vi "Test GUI.vi"() -> ()   [LabVIEW 2018]
doc: "Acoustic Test for EOL"
uses:
  Types/EnumType.ctl
  <vilib>/Utility/miscctls.llb/LVRowAndColumnTypeDef.ctl
  <vilib>/Utility/miscctls.llb/LVRowAndColumnUnsignedTypeDef.ctl
  <vilib>/Utility/error.llb/DialogType.ctl
  Supports/Global 1.vi
panel:
  out "1.6 part":bool
  out "1.7 part":bool
  out "ME79 MODEL":enum16{"E183362", "E180639", "E415025"}(ring)
  out "SN":u16
  in  "ZEBRA PRINT ME74":bool
  in  "Reset Conter 2":bool
  out "TARGET COUNTER":dbl
  in  "PLAN TARGET":dbl
  out "CounterFull 2":bool
  out "Buffer 2":u16
  out "Buffer":u16
  out "MIC 2":cluster{dbl[], dbl[]}[](graph)
  out "Test Data":string[][](table)
  out "MIC 1":cluster{dbl[], dbl[]}[](graph)
  in  "Change Model":bool
  in  "Alarm":u16
  out "Alarm Display":string
  out "MCError":bool
  out "Auto Running":bool
  out "CYCLE\nTIME":u16
  in  "Reset Conter":bool
  out "NG":dbl
  out "OK":dbl
  in  "BOX TARGET":dbl
  out "CounterFull":bool
  out "File Open Reference out":T1
  out "Test Error":bool
  out "Power OK":bool
  in  "Print":bool=TRUE
  out "LBL Data":T2
  in  "Cal Mic CH":bool
  out "AT Cond 2":bool
  out "AT Cond":bool
  in  "IAI Cal":bool
  in  "IAI Ret":bool
  in  "IAI Adv":bool
  out "Status":string
  in  "Calibrate":bool
  out "Connection":bool
  out "Stop":bool
  out "Start":bool
  out "Error":bool
  out "Fail":bool
  out "Pass":bool
  out "Done":bool
  out "Busy":bool
  out "Ready":bool
  in  "Channel":bool
  out "Model":bool
  in  "Start":bool
  in  "Mode":bool
  in  "Quit":bool
  out "Test Result":bool
  out "Test Running":bool
  # "MICROPHONE TEST EOL"
  # "TEST DATA"
  # "MANUAL CONTROL"
  # "BUFFER\nE180639"
  # "BUFFER\nE183362"
  # "Version 3.1 Build 20200630"
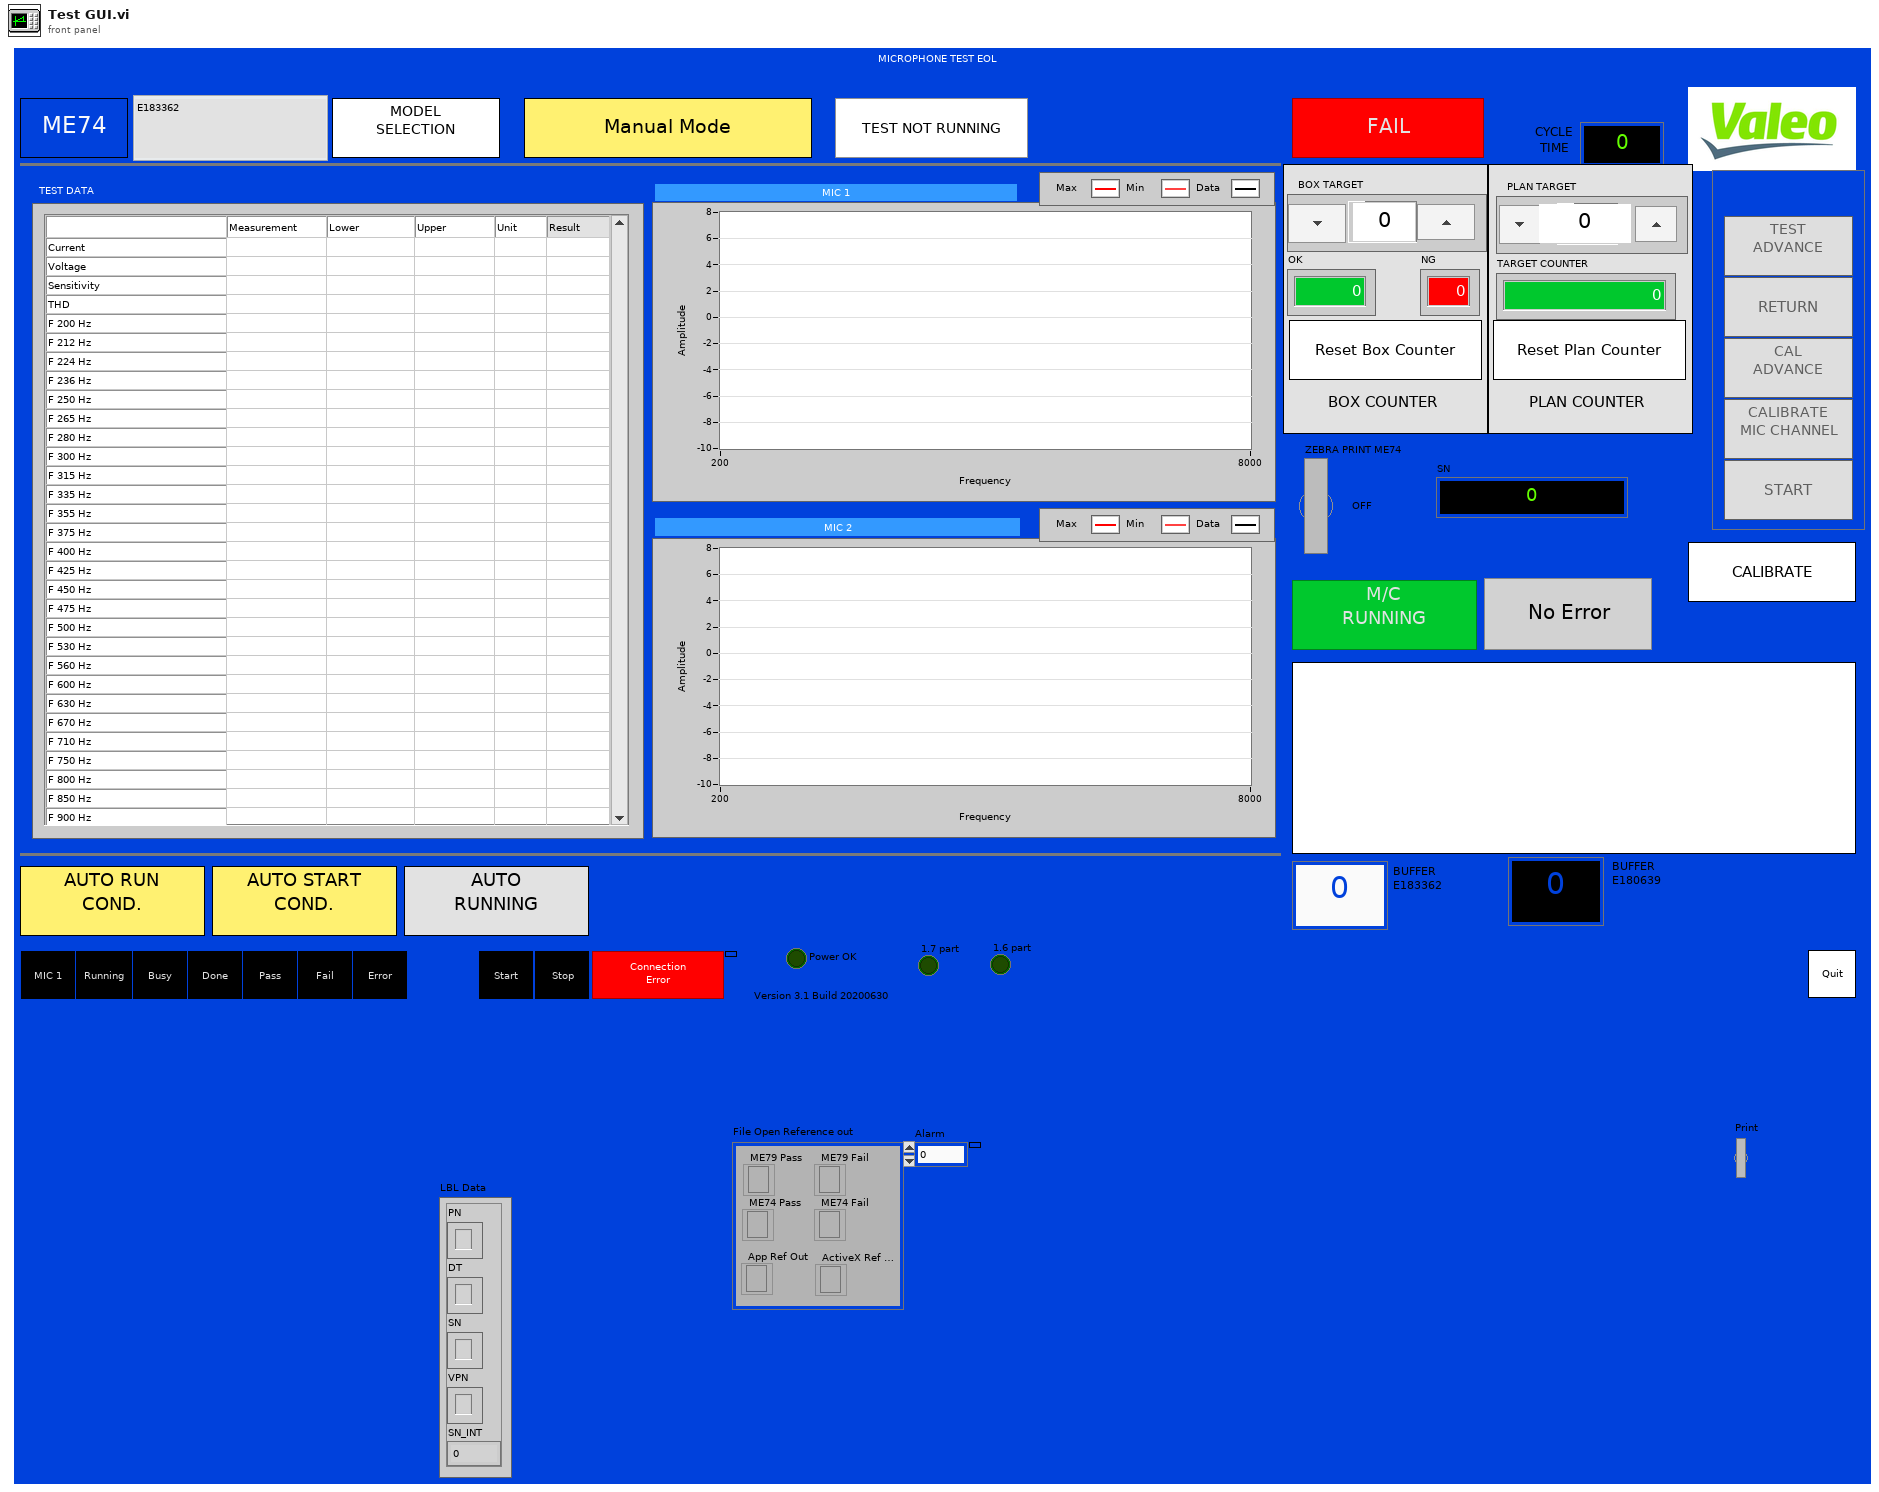
[diagram p1: front panel]
types:
  T1 = cluster{"ME79 Pass":refnum<k7>, "ME79 Fail":refnum<k7>, "ME74 Pass":refnum<k7>, "ME74 Fail":refnum<k7>, "App Ref Out":refnum<k7>, "ActiveX Ref Out":refnum<k7>}
  T2 = cluster{"PN":string, "DT":string, "SN":string, "VPN":string, "SN_INT":i32}
  T3 = typedef "EnumType.ctl" = enum16{"Initial", "Wait PLC Connect", "Ready", "Load and Init Config", "Power Supply On", "Freq Sweep 1", "Freq Sweep 2", "Power Supply Off", "Save Test Data", "Print Label", "Display Result", "Quit", "Calibration"}
  T4 = enum8{"Enabled", "Disabled", "Disabled and Grayed Out"}
  T5 = typedef "LVRowAndColumnTypeDef.ctl" = cluster{"Row":i32, "Column":i32}
  T6 = typedef "LVRowAndColumnUnsignedTypeDef.ctl" = cluster{"Row":u32, "Column":u32}
  T7 = typedef "LimitType.ctl" = cluster{"PSU":cluster{"Current Lower (mA)":dbl, "Current Upper (mA)":dbl, "Voltage Lower (V)":dbl, "Voltage Upper (V)":dbl}, "Mic":cluster{"Sensitivity (mV/Pa)":cluster{"Lower":dbl, "Upper":dbl}, "THD (%)":cluster{"Lower":dbl, "Upper":dbl}, "Freq Response":cluster{"Freq":dbl, "Upper":dbl, "Lower":dbl}[]}}
  T8 = typedef "ConfigurationType.ctl" = cluster{"PSU Setting":T9, "Sweep Settings":T10}
  T9 = typedef "SupplyConfig.ctl" = cluster{"Channel Name":string, "Source Delay (Sec)":dbl, "Measurement:Sense":i32, "voltage level":dbl, "voltage level range":dbl, "current limit":dbl, "current limit range":dbl, "resource name":refnum<k15>}
  T10 = typedef "Peiker_Stepped Sweep Settings.ctl" = cluster{"Input Settings":cluster{"IEPE min time to settle [s]":dbl, "Responce Channel Settings":cluster{"DSA response channel settings":T11, "response channel info":T12, "AI response settings":cluster{"response channel":tag, "max value [V]":dbl, "min value [V]":dbl, "terminal configuration":i32}}, "Stimulus Channel Settings":cluster{"AI stimulus settings":cluster{"stimulus channel":tag, "max value [V]":dbl, "min value [V]":dbl, "terminal configuration":i32}, "DSA stimulus channel settings":T11, "stimulus channel info":T12}}, "Output Settings":cluster{"AO source settings":cluster{"excitation channel":tag, "max value [V]":dbl, "min value [V]":dbl, "terminal configuration":i32}}}
  T11 = typedef "svc_DSA Channel Settings.ctl" = cluster{"coupling":i32, "enable IEPE excitation":bool, "IEPE current [mA]":dbl}
  T12 = typedef "svc_Channel Info.ctl" = cluster{"sensor sensitivity":dbl, "engineering units":T13, "dB reference":dbl, "custom label":string, "weighting filter":T14, "pregain":dbl}
  T13 = typedef "svc_Engineering Units Text Ring.ctl" = u16
  T14 = typedef "svc_Weighting Filter Text Ring.ctl" = u16
  T15 = cluster{"Label Data":string, "Label Data":string, "Label Data":string, "Label Data":string, "Cycle Time (ms)":i32}
  T16 = typedef "DialogType.ctl" = u16
  T17 = cluster{"frequency [Hz]":dbl[], "amplitude":dbl[]}
  T18 = cluster{string, "DT":string, "SN":string, "date/time string":string, "LINECODE":string, "NG CODE OUT":string}
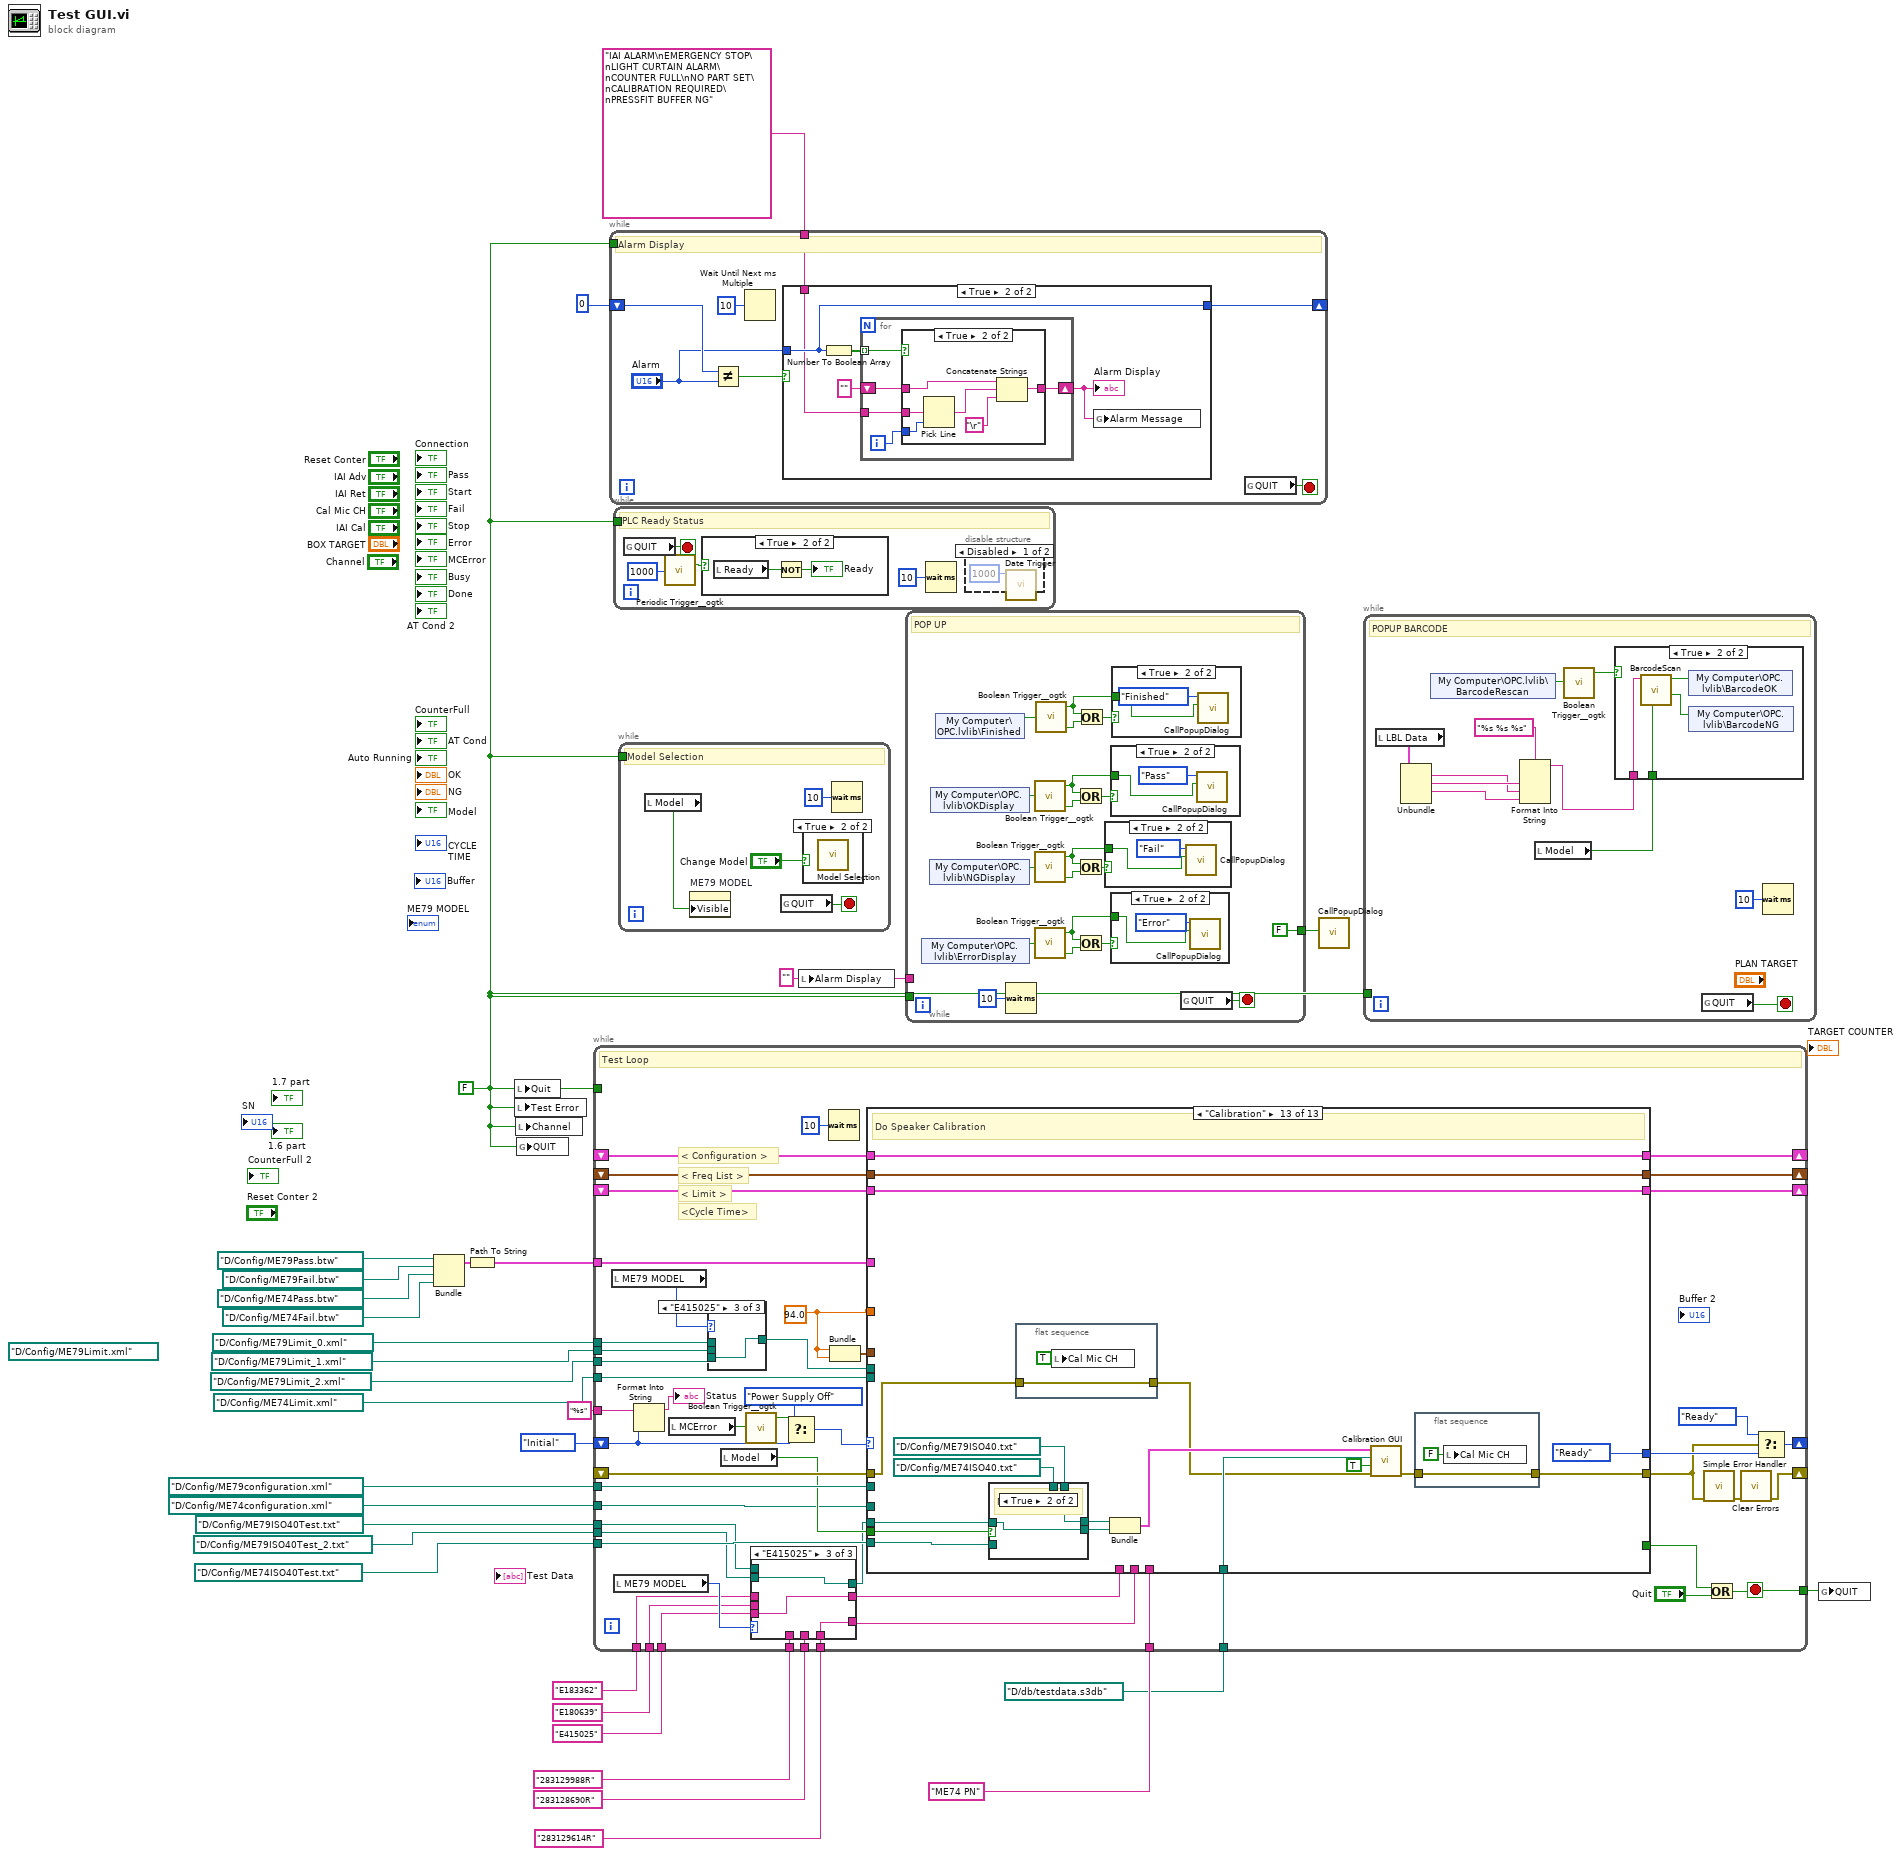
[diagram p0: block diagram]
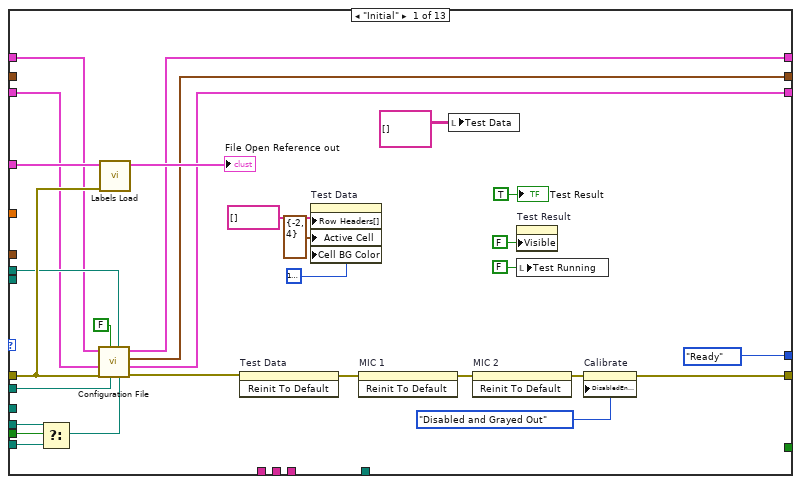
[diagram p16: hidden frame]
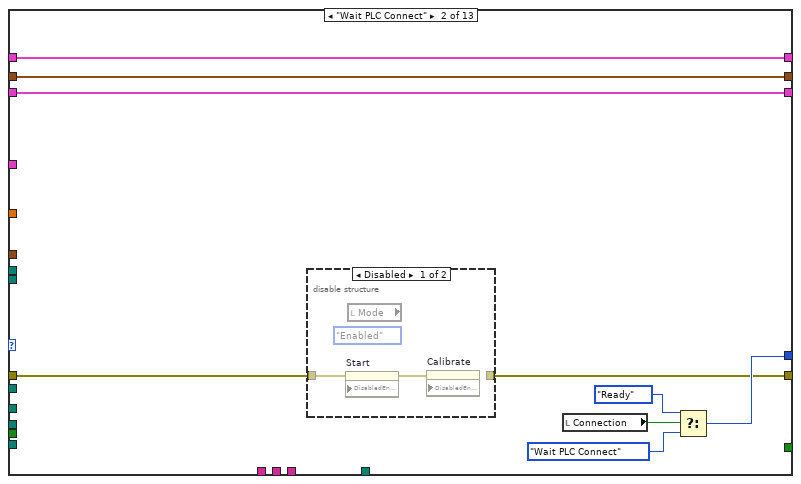
[diagram p17: hidden frame]
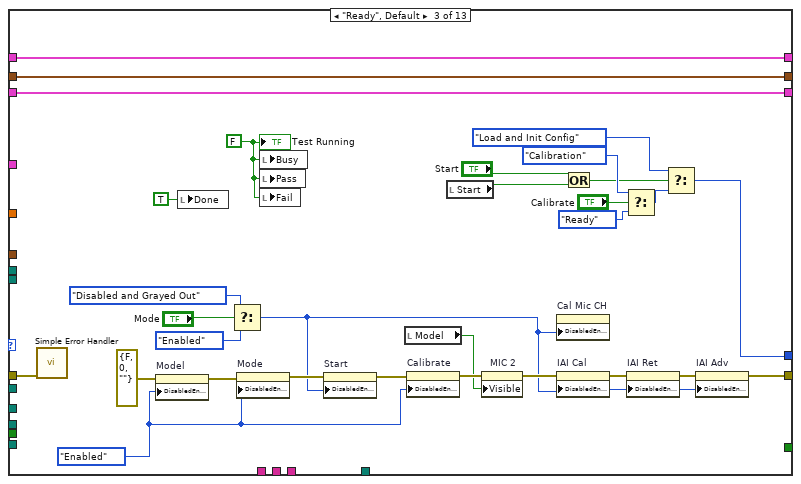
[diagram p19: hidden frame]
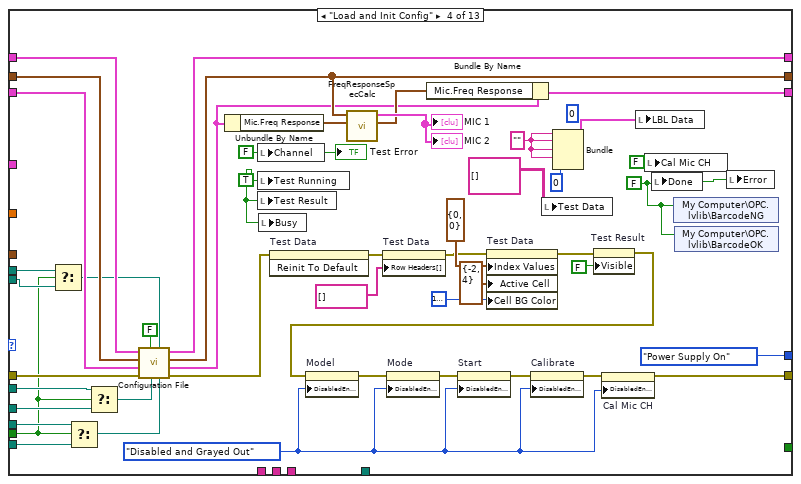
[diagram p20: hidden frame]
diagram:
  (unwired) path "D:/Config/ME79Limit.xml"
  w11 = ""
  w10 = FALSE ("Quit")
  n1 = Bundle(path "D:/Config/ME79Pass.btw", path "D:/Config/ME79Fail.btw", path "D:/Config/ME74Pass.btw", path "D:/Config/ME74Fail.btw") -> (w28:cluster{path, path, path, path})  [unwired: 1 in]
  n2 = Path To String(path=w28) -> (string=w29:cluster{string, string, string, string})
  n3 = local write "Quit"(w10) -> ()
  n4 = local write "Test Error"(w10) -> ()
  n5 = local write "Channel"(w10) -> ()
  n6 = global write "Global 1.vi" "QUIT"(w10) -> ()
  n7 = while {
    shift-right: [w71] -> _
    shift-left: EnumType."Initial" ("Enum") -> [w57]
    shift-right: [w69] -> _
    shift-left: _ -> [w81]
    tunnel: path "D:/Config/ME79configuration.xml" -> [w80]
    shift-right: [w79] -> _
    shift-left: _ -> [w78]
    shift-right: [w76] -> _
    shift-left: _ -> [w77]
    tunnel: path "D:/Config/ME79ISO40Test.txt" -> [w32]
    shift-right: [w74] -> _
    shift-left: _ -> [w75]
    tunnel: path "D:/Config/ME79Limit_0.xml" -> [w38]
    tunnel: path "D:/db/testdata.s3db" -> [w68]
    tunnel: path "D:/Config/ME74ISO40Test.txt" -> [w66]
    tunnel: w10 -> [_]
    tunnel: "ME74 PN" -> [w63]
    tunnel: w29 -> [w60]
    tunnel: "E183362" -> [w47]
    tunnel: "E180639" -> [w46]
    tunnel: "283129988R" -> [w42]
    tunnel: "283128690R" -> [w41]
    tunnel: path "D:/Config/ME74configuration.xml" -> [w53]
    tunnel: path "D:/Config/ME74Limit.xml" -> [w52]
    tunnel: "%s" ("format string") -> [w50]
    tunnel: [w49] -> w12
    tunnel: "E415025" -> [w45]
    tunnel: "283129614R" -> [w40]
    tunnel: path "D:/Config/ME79Limit_1.xml" -> [w37]
    tunnel: path "D:/Config/ME79Limit_2.xml" -> [w36]
    tunnel: path "D:/Config/ME79ISO40Test_2.txt" -> [w34]
    stop <- w49 stop-if-true
    w59 = 94.0 ("dB Reference")
    # "<Cycle Time>"
    # "< Limit >"
    # "< Freq List >"
    # "< Configuration >"
    # "Test Loop"
    n8 = local read "ME79 MODEL"() -> (w35:enum16{"E183362", "E180639", "E415025"})
    n9 = local read "ME79 MODEL"() -> (w48:enum16{"E183362", "E180639", "E415025"})
    n10 = Format Into String(format string=w50, w57) -> (resulting string=→"Status":string)  [unwired: 2 in, 1 out]
    n11 = local read "MCError"() -> (w55:bool)
    n12 = case shown="\"E415025\"" w35 {
      tunnel: [w83 w84 w85] -> w39
      tunnel: w38 -> [w83 _ _]
      tunnel: w37 -> [_ w84 _]
      tunnel: w36 -> [_ _ w85]
      frame "E183362", Default {
      }
      frame "E180639" {
      }
      frame "E415025" {
      }
    }
    n13 = local read "Model"() -> (w67:bool)
    n14 = call <userlib>:"Boolean Trigger__ogtk.vi"("Boolean Input"=w55) -> ("Rising Edge"=w54:bool)  [unwired: 1 in, 1 out]
    n15 = case shown="\"E415025\"" w48 {
      tunnel: w47 -> [w88 _ _]
      tunnel: w46 -> [_ w91 _]
      tunnel: w45 -> [_ _ w94]
      tunnel: [w88 w91 w94] -> w44
      tunnel: w42 -> [w87 _ _]
      tunnel: [w87 w90 w93] -> w43
      tunnel: w41 -> [_ w90 _]
      tunnel: w40 -> [_ _ w93]
      tunnel: w34 -> [_ _ w92]
      tunnel: [w86 w89 w92] -> w33
      tunnel: w32 -> [w86 w89 _]
      frame "E183362", Default {
      }
      frame "E180639" {
      }
      frame "E415025" {
      }
    }
    n16 = Select(t=EnumType."Power Supply Off" ("Enum"), s=w54, f=w57) -> (s? t:f=w56:T3)
    n17 = Wait (ms)(milliseconds to wait=u32 10) -> ()  [unwired: 1 out]
    n18 = Bundle("dB Reference"=w59, "dB Reference"=w59) -> (w62:cluster{"dB Reference":dbl, "dB Reference":dbl})  [unwired: 1 in]
    n19 = case shown="\"Calibration\"" w56 {
      tunnel: w81 -> [w108 w125 w162 w211 w238 w262 w294 w323 w354 w383 w417 w450 w457]
      tunnel: [w113 w124 w142 w179 w217 w242 w292 w325 w350 w397 w418 w450 w454] -> w61
      tunnel: [EnumType."Ready" ("Enum") w131 w157 EnumType."Power Supply On" ("Enum") w229 w245 EnumType."Power Supply Off" ("Enum") w315 EnumType."Print Label" ("Enum") EnumType."Display Result" ("Enum") EnumType."Ready" ("Enum") EnumType."Quit" ("Enum") EnumType."Ready" ("Enum")] -> w73
      tunnel: [_ _ _ _ _ _ _ _ _ _ _ TRUE _] -> w65
      tunnel: w80 -> [w106 _ _ w173 _ _ _ _ _ _ _ _ _]
      tunnel: [w99 w130 w165 w209 w222 w271 w303 w327 w357 w401 w422 w448 w465] -> w79
      tunnel: w78 -> [w98 w130 w165 w208 w222 w271 w303 w327 w357 w401 w422 w448 w465]
      tunnel: [w97 w129 w164 w186 w216 w248 w301 w329 w333 w400 w421 w447 w466] -> w76
      tunnel: w77 -> [_ w129 w164 w207 w216 w248 w301 w329 w333 w400 w421 w447 w466]
      tunnel: w33 -> [w104 _ _ w199 _ _ _ _ _ _ _ _ w462]
      tunnel: w75 -> [w95 w128 w163 w206 w215 w251 w282 w328 w356 w399 w420 w446 w467]
      tunnel: [w96 w128 w163 w202 w215 w251 w282 w328 w356 w399 w420 w446 w467] -> w74
      tunnel: w39 -> [w101 _ _ w171 _ _ _ _ _ _ _ _ _]
      tunnel: w68 -> [_ _ _ _ _ _ _ _ w353 _ _ _ w458]
      tunnel: w67 -> [w105 _ _ w169 _ w239 w275 _ w331 w375 _ _ w464]
      tunnel: w66 -> [w103 _ _ w198 _ _ _ _ _ _ _ _ w461]
      tunnel: w62 -> [_ _ _ _ _ w257 w288 _ _ _ _ _ _]
      tunnel: w59 -> [_ _ _ _ _ w256 w287 _ _ _ _ _ _]
      tunnel: w44 -> [_ _ _ _ _ _ _ _ w347 w377 _ _ _]
      tunnel: w63 -> [_ _ _ _ _ _ _ _ w346 _ _ _ _]
      tunnel: w60 -> [w110 _ _ _ _ _ _ _ _ _ _ _ _]
      tunnel: w43 -> [_ _ _ _ _ _ _ _ _ w378 _ _ _]
      tunnel: w53 -> [_ _ _ w174 _ _ _ _ _ _ _ _ _]
      tunnel: w52 -> [_ _ _ w170 _ _ _ _ _ _ _ _ _]
      frame "Initial" {
        n20 = Select(t=w104, s=w105, f=w103) -> (s? t:f=w102:path)
        n21 = call "Configuration File.vi"("Freq List File"=w102, "Limit File"=w101, "Configurtion File"=w106, "Mode (F-Read)"=FALSE, "Error In"=w108, "Limit"=w95, "Configuration"=w98) -> ("Error Out"=w107:errorcluster, "Limit Out"=w96:T7, "Freq List Out"=w97:cluster{"Freq":dbl, "Amp":dbl}[], "value"=w99:T8)  [unwired: 1 in]
        n22 = call "Labels Load.vi"("error in (no error)"=w108, "Labels"=w110) -> ("File Open Reference out"=→"File Open Reference out":T1)  [unwired: 8 in, 1 out]
        n23 = invoke on="Test Data" class="Tbl (strict)" method="Reinit To Default"(error in=w107) -> (error out=w121:errorcluster)  [unwired: 2 in, 2 out]
        n24 = property on="Test Data" class="Tbl (strict)"("Row Headers[]"=string[] [], "Active Cell"=T5 {"Row"=-2, "Column"=4} ("Active Cell:Active Cell"), "Cell BG Color"=u32 16777225) -> ()  [unwired: 2 in, 2 out]
        n25 = invoke on="MIC 1" class="XYGraph (strict)" method="Reinit To Default"(error in=w121) -> (error out=w120:errorcluster)  [unwired: 2 in, 2 out]
        n26 = local write "Test Data"(string[][] []) -> ()
        n27 = invoke on="MIC 2" class="XYGraph (strict)" method="Reinit To Default"(error in=w120) -> (error out=w114:errorcluster)  [unwired: 2 in, 2 out]
        n28 = property on="Test Result" class="Bool (strict)"("Visible"=FALSE) -> ()  [unwired: 2 in, 2 out]
        n29 = local write "Test Running"(FALSE ("Test Running")) -> ()
        n30 = property on="Calibrate" class="Bool"(error in=w114, "DisabledEnum"=T4."Disabled and Grayed Out" ("Disabled")) -> (error out=w113:errorcluster)  [unwired: 1 in, 1 out]
        "Test Result" <- TRUE ("Test Pass")
      }
      frame "Wait PLC Connect" {
        n31 = disable-structure shown="Disabled" {
          disable-tunnel: w125 -> [w134 w135]
          disable-tunnel: [_ w135] -> w124
          frame Disabled {
            (unwired) T4."Enabled" ("Disabled")
            n32 = property on="Start" class="Bool (strict)" props=["DisabledEnum"](error in=w134) -> (error out=w133:errorcluster)  [unwired: 2 in, 1 out]
            n33 = local read "Mode"() -> ()  [unwired: 1 out]
            n34 = property on="Calibrate" class="Bool" props=["DisabledEnum"](error in=w133) -> ()  [unwired: 2 in, 2 out]
          }
          frame Enabled {
          }
        }
        n35 = local read "Connection"() -> (w132:bool)
        n36 = Select(t=EnumType."Ready" ("Enum"), s=w132, f=EnumType."Wait PLC Connect" ("Enum")) -> (s? t:f=w131:T3)
      }
      frame "Ready", Default {
        w147 = T4."Enabled" ("Disabled")
        w139 = FALSE ("Test Running")
        n37 = call <vilib>:"Simple Error Handler.vi"("error in (no error)"=w162) -> ()  [unwired: 4 in, 5 out]
        n38 = property on="Model" class="Bool (strict)"(error in=errorcluster {"status"=FALSE, "code"=0, "source"=""} ("Error Out"), "DisabledEnum"=w147) -> (error out=w151:errorcluster)  [unwired: 1 in, 1 out]
        n39 = local write "Done"(TRUE ("Done")) -> ()
        n40 = Select(t=T4."Disabled and Grayed Out" ("Disabled"), s="Mode", f=T4."Enabled" ("Disabled")) -> (s? t:f=w138:T4)
        n41 = property on="Mode" class="Bool (strict)"(error in=w151, "DisabledEnum"=w147) -> (error out=w150:errorcluster)  [unwired: 1 in, 1 out]
        n42 = local write "Busy"(w139) -> ()
        n43 = local write "Pass"(w139) -> ()
        n44 = local write "Fail"(w139) -> ()
        n45 = property on="Start" class="Bool (strict)"(error in=w150, "DisabledEnum"=w138) -> (error out=w148:errorcluster)  [unwired: 1 in, 1 out]
        n46 = local read "Model"() -> (w136:bool)
        n47 = property on="Calibrate" class="Bool"(error in=w148, "DisabledEnum"=w147) -> (error out=w146:errorcluster)  [unwired: 1 in, 1 out]
        n48 = local read "Start"() -> (w137:bool)
        n49 = property on="MIC 2" class="XYGraph (strict)"(error in=w146, "Visible"=w136) -> (error out=w143:errorcluster)  [unwired: 1 in, 1 out]
        n50 = property on="Cal Mic CH" class="Bool (strict)"("DisabledEnum"=w138) -> ()  [unwired: 2 in, 2 out]
        n51 = property on="IAI Cal" class="Bool (strict)"(error in=w143, "DisabledEnum"=w138) -> (error out=w145:errorcluster)  [unwired: 1 in, 1 out]
        n52 = Or(x="Start", y=w137) -> (x .or. y?=w153:bool)
        n53 = Select(t=EnumType."Calibration" ("Enum"), s="Calibrate", f=EnumType."Ready" ("Enum")) -> (s? t:f=w158:T3)
        n54 = property on="IAI Ret" class="Bool (strict)"(error in=w145, "DisabledEnum"=w138) -> (error out=w144:errorcluster)  [unwired: 1 in, 1 out]
        n55 = Select(t=EnumType."Load and Init Config" ("Enum"), s=w153, f=w158) -> (s? t:f=w157:T3)
        n56 = property on="IAI Adv" class="Bool (strict)"(error in=w144, "DisabledEnum"=w138) -> (error out=w142:errorcluster)  [unwired: 1 in, 1 out]
        "Test Running" <- w139
      }
      frame "Load and Init Config" {
        w175 = "" ("Label Data")
        w167 = FALSE ("Done")
        (unwired) 0 ("Cycle Time (ms)")
        w176 = FALSE ("Channel")
        w182 = TRUE ("Test Running")
        w178 = T4."Disabled and Grayed Out" ("Disabled")
        n57 = Select(t=w171, s=w169, f=w170) -> (s? t:f=w168:path)
        n58 = Select(t=w199, s=w169, f=w198) -> (s? t:f=w197:path)
        n59 = Select(t=w173, s=w169, f=w174) -> (s? t:f=w172:path)
        n60 = call "Configuration File.vi"("Freq List File"=w197, "Limit File"=w168, "Configurtion File"=w172, "Mode (F-Read)"=FALSE, "Error In"=w211, "Limit"=w206, "Freq List In"=w207, "Configuration"=w208) -> ("Error Out"=w194:errorcluster, "Limit Out"=w185:T7, "Freq List Out"=w186:cluster{"Freq":dbl, "Amp":dbl}[], "value"=w209:T8)
        n61 = Unbundle By Name(w185) -> ("Mic.Freq Response"=w205:cluster{"Freq":dbl, "Upper":dbl, "Lower":dbl}[])
        n62 = local write "Channel"(w176) -> ()
        n63 = local write "Test Running"(w182) -> ()
        n64 = local write "Test Result"(w182) -> ()
        n65 = local write "Busy"(w182) -> ()
        n66 = invoke on="Test Data" class="Tbl (strict)" method="Reinit To Default"(error in=w194) -> (error out=w200:errorcluster)  [unwired: 2 in, 2 out]
        n67 = call "FreqResponseSpecCalc.vi"("Freq Response Spec In"=w205, "Freq List In"=w186) -> ("All Freq Spec Out"=w203:cluster{"Freq":dbl, "Upper":dbl, "Lower":dbl}[], "XY Graph"=→"MIC 1" →"MIC 2":cluster{dbl[], dbl[]}[])  [unwired: 8 in]
        n68 = property on="Test Data" class="Tbl (strict)"(error in=w200, "Row Headers[]"=string[] [] ("Row Header Strings[]")) -> (error out=w195:errorcluster)  [unwired: 1 in, 1 out]
        n69 = Bundle By Name(cluster=w185, "Mic.Freq Response"=w203) -> (w202:T7)
        n70 = property on="Test Data" class="Tbl (strict)"(error in=w195, "Index Values"=T6 {"Row"=0, "Column"=0}, "Active Cell"=T5 {"Row"=-2, "Column"=4} ("Active Cell:Active Cell"), "Cell BG Color"=u32 16777225) -> (error out=w184:errorcluster)  [unwired: 1 in, 1 out]
        n71 = local write "Test Data"(string[][] []) -> ()
        n72 = Bundle("Label Data"=w175, "Label Data"=w175, "Label Data"=w175, "Label Data"=w175, "Cycle Time (ms)"=0) -> (w177:T15)  [unwired: 1 in]
        n73 = property on="Test Result" class="Bool (strict)"(error in=w184, "Visible"=FALSE) -> (error out=w183:errorcluster)  [unwired: 1 in, 1 out]
        n74 = property on="Model" class="Bool (strict)"(error in=w183, "DisabledEnum"=w178) -> (error out=w192:errorcluster)  [unwired: 1 in, 1 out]
        n75 = property on="Mode" class="Bool (strict)"(error in=w192, "DisabledEnum"=w178) -> (error out=w191:errorcluster)  [unwired: 1 in, 1 out]
        n76 = property on="Start" class="Bool (strict)"(error in=w191, "DisabledEnum"=w178) -> (error out=w188:errorcluster)  [unwired: 1 in, 1 out]
        n77 = property on="Calibrate" class="Bool"(error in=w188, "DisabledEnum"=w178) -> (error out=w180:errorcluster)  [unwired: 1 in, 1 out]
        n78 = property on="Cal Mic CH" class="Bool (strict)"(error in=w180, "DisabledEnum"=w178) -> (error out=w179:errorcluster)  [unwired: 1 in, 1 out]
        n79 = local write "LBL Data"(w177) -> ()
        n80 = local write "Cal Mic CH"(FALSE ("IAI Cal 2")) -> ()
        n81 = local write "Done"(w167) -> ()
        n82 = shared-variable "My Computer\\OPC.lvlib\\BarcodeNG"(w167) -> ()  [unwired: 1 in, 1 out]
        n83 = shared-variable "My Computer\\OPC.lvlib\\BarcodeOK"(w167) -> ()  [unwired: 1 in, 1 out]
        n84 = local write "Error"(w167) -> ()
        "Test Error" <- w176
      }
      frame "Power Supply On" {
        n85 = Unbundle By Name(w222) -> ("PSU Setting"=w221:T9)
        n86 = Unbundle By Name(w215) -> ("PSU.Current Upper (mA)"=w237:dbl, "PSU.Current Lower (mA)"=w236:dbl, "PSU.Voltage Upper (V)"=w235:dbl, "PSU.Voltage Lower (V)"=w234:dbl)
        n87 = call "PSU ON.vi"("Error In"=w238, "PSU Setting"=w221) -> ("Error Out"=w228:errorcluster, "Current Result (mA)"=w227:dbl, "Volt Result"=w226:dbl)  [unwired: 6 in, 1 out]
        n88 = local read "Test Result"() -> (w224:bool)
        n89 = control-ref of="Test Data"() -> (w219:refnum<vi>)
        n90 = Build Array(w227, w226) -> (w225:dbl[])
        n91 = In Range and Coerce(upper limit=w237, x=w227, lower limit=w236) -> (In Range?=w233:bool)  [unwired: 1 out]
        n92 = In Range and Coerce(upper limit=w235, x=w226, lower limit=w234) -> (In Range?=w232:bool)  [unwired: 1 out]
        n93 = call "Update Test Data Table.vi"("Enum"=enum16{"PSU", "Mic"}."PSU", "Prev Result in"=w224, "Error In"=w228, "Test Data In"=w225, "Limit In"=w215, "Test Data ref in"=w219) -> ("Error Out"=w220:errorcluster, "Latest Result Out"=w214:bool)  [unwired: 4 in]
        n94 = And(x=w233, y=w232) -> (x .and. y?=w213:bool)
        "Power OK" <- w213
        n95 = local write "Test Result"(w214) -> ()
        n96 = call "Table Result Color.vi"("Error In"=w220, "Result Column"=4, "Table Ref"=w219) -> ("Error Out"=w217:errorcluster)  [unwired: 8 in]
        n97 = Select(t=EnumType."Freq Sweep 1" ("Enum"), s=w213, f=EnumType."Power Supply Off" ("Enum")) -> (s? t:f=w229:T3)
      }
      frame "Freq Sweep 1" {
        w240 = T16 0 items=["no dialog", "OK message", "continue or stop message", "OK message + warnings", "continue/stop + warnings"] ("type of dialog (OK msg:1)")
        n98 = stacked-sequence {
          tunnel: w262 -> [_ w274]
          tunnel: [_ w273] -> w261
          frame #0 {
            n99 = local write "Channel"(FALSE) -> ()
          }
          frame #1 {
            n100 = call "Time Delay2"("error in (no error)"=w274) -> ("error out"=w273:errorcluster)  [unwired: 10 in]
          }
        }
        n101 = Unbundle By Name(w251) -> ("Mic.Freq Response"=w250:cluster{"Freq":dbl, "Upper":dbl, "Lower":dbl}[])
        n102 = Unbundle By Name(w271) -> ("Sweep Settings"=w270:T10)
        n103 = local read "Test Result"() -> (w265:bool)
        n104 = local read "MIC 1"() -> (w254:cluster{dbl[], dbl[]}[])
        n105 = call "Single Mic Test.vi"("Peiker_Stepped Sweep Settings"=w270, "Freq Response Limit"=w250, "frequency list Input"=w248, "Error In"=w261, "Test Level"=w257, "Model (T-79)"=w239, "dB Reference"=w256, "String"="SW1.txt") -> ("Processed Freq Response"=w253:T17, "Test Result Out"=w266:dbl[], "Error Out"=w264:errorcluster)  [unwired: 4 in, 1 out]
        n106 = Insert Into Array(array=w254, new element=w253) -> (w252:cluster{dbl[], dbl[]}[])  [unwired: 1 in]
        n107 = control-ref of="Test Data"() -> (w259:refnum<vi>)
        n108 = call "Update Test Data Table.vi"("Enum"=enum16{"PSU", "Mic"}."Mic", "Prev Result in"=w265, "Error In"=w264, "Test Data In"=w266, "Limit In"=w251, "Test Data ref in"=w259) -> ("Error Out"=w260:errorcluster, "Latest Result Out"=w249:bool)  [unwired: 4 in]
        n109 = local write "MIC 1"(w252) -> ()
        n110 = call "Table Result Color.vi"("Error In"=w260, "Result Column"=4, "Table Ref"=w259) -> ("Error Out"=w244:errorcluster)  [unwired: 8 in]
        n111 = local write "Test Result"(w249) -> ()
        n112 = call <vilib>:"Simple Error Handler.vi"("type of dialog (OK msg:1)"=w240, "error in (no error)"=w244) -> ("error?"=w241:bool, "error out"=w243:errorcluster)  [unwired: 3 in, 3 out]
        n113 = local read "Model"() -> (w269:bool)
        n114 = local write "Test Error"(w241) -> ()
        n115 = call <userlib>:"Clear All Errors__ogtk.vi"("Error In"=w243) -> ("Error Out"=w242:errorcluster)  [unwired: 3 in]
        n116 = Select(t=EnumType."Freq Sweep 2" ("Enum"), s=w269, f=EnumType."Power Supply Off" ("Enum")) -> (s? t:f=w246:T3)
        n117 = local write "Error"(w241) -> ()
        n118 = Select(t=EnumType."Power Supply Off" ("Enum"), s=w244, f=w246) -> (s? t:f=w245:T3)
      }
      frame "Freq Sweep 2" {
        w276 = T16 0 items=["no dialog", "OK message", "continue or stop message", "OK message + warnings", "continue/stop + warnings"] ("type of dialog (OK msg:1)")
        n119 = stacked-sequence {
          tunnel: w294 -> [_ w310]
          tunnel: [_ w309] -> w293
          frame #0 {
            n120 = local write "Channel"(TRUE) -> ()
          }
          frame #1 {
            n121 = call "Time Delay"("error in (no error)"=w310) -> ("error out"=w309:errorcluster)  [unwired: 10 in]
          }
        }
        n122 = Unbundle By Name(w303) -> ("Sweep Settings"=w302:T10)
        n123 = Unbundle By Name(w282) -> ("Mic.Freq Response"=w281:cluster{"Freq":dbl, "Upper":dbl, "Lower":dbl}[])
        n124 = local read "Test Result"() -> (w296:bool)
        n125 = local read "MIC 2"() -> (w285:cluster{dbl[], dbl[]}[])
        n126 = call "Single Mic Test.vi"("Peiker_Stepped Sweep Settings"=w302, "Freq Response Limit"=w281, "frequency list Input"=w301, "Error In"=w293, "Test Level"=w288, "Model (T-79)"=w275, "dB Reference"=w287, "String"="SW2.txt") -> ("Processed Freq Response"=w284:T17, "Test Result Out"=w297:dbl[], "Error Out"=w298:errorcluster)  [unwired: 4 in, 1 out]
        n127 = control-ref of="Test Data"() -> (w291:refnum<vi>)
        n128 = Insert Into Array(array=w285, new element=w284) -> (w283:cluster{dbl[], dbl[]}[])  [unwired: 1 in]
        n129 = call "Update Test Data Table.vi"("Enum"=enum16{"PSU", "Mic"}."Mic", "Prev Result in"=w296, "Error In"=w298, "Test Data In"=w297, "Limit In"=w282, "Test Data ref in"=w291) -> ("Error Out"=w289:errorcluster, "Latest Result Out"=w295:bool)  [unwired: 4 in]
        n130 = local write "MIC 2"(w283) -> ()
        n131 = call "Table Result Color.vi"("Error In"=w289, "Result Column"=4, "Table Ref"=w291) -> ("Error Out"=w280:errorcluster)  [unwired: 8 in]
        n132 = local write "Test Result"(w295) -> ()
        n133 = call <vilib>:"Simple Error Handler.vi"("type of dialog (OK msg:1)"=w276, "error in (no error)"=w280) -> ("error?"=w277:bool, "error out"=w279:errorcluster)  [unwired: 3 in, 3 out]
        n134 = call <userlib>:"Clear All Errors__ogtk.vi"("Error In"=w279) -> ("Error Out"=w278:errorcluster)  [unwired: 3 in]
        n135 = local write "Test Error"(w277) -> ()
        n136 = stacked-sequence {
          tunnel: w278 -> [_ w307]
          tunnel: [_ w306] -> w292
          frame #0 {
            n137 = local write "Channel"(FALSE) -> ()
          }
          frame #1 {
            n138 = call "Time Delay3"("error in (no error)"=w307, "Delay Time (s)"=0.2) -> ("error out"=w306:errorcluster)  [unwired: 9 in]
          }
        }
        n139 = local write "Error"(w277) -> ()
      }
      frame "Power Supply Off" {
        n140 = Unbundle By Name(w327) -> ("PSU Setting.resource name"=w311:refnum<k15>)
        n141 = property on="Test Result" class="Bool (strict)"(error in=w323, "Visible"=TRUE) -> (error out=w322:errorcluster)  [unwired: 1 in, 1 out]
        n142 = control-ref of="Test Data"() -> (w319:refnum<vi>)
        n143 = call "Reset_Power_Supply.vi"("error in (no error)"=errorcluster {"status"=FALSE, "code"=0, "source"=""}, "resource name"=w311) -> ("error out"=w321:errorcluster)  [unwired: 9 in]
        n144 = call "Table Result Color.vi"("Error In"=w321, "Result Column"=4, "Table Ref"=w319) -> ("Error Out"=w320:errorcluster)  [unwired: 8 in]
        n145 = Merge Errors(w322, w320) -> (w325:errorcluster)
        n146 = local read "MCError"() -> (w314:bool)
        n147 = local read "Test Error"() -> (w313:bool)
        n148 = Or(x=w314, y=w313) -> (x .or. y?=w312:bool)
        n149 = Select(t=EnumType."Display Result" ("Enum"), s=w312, f=EnumType."Save Test Data" ("Enum")) -> (s? t:f=w315:T3)
      }
      frame "Save Test Data" {
        (unwired) string[] [] ("f")
        n150 = local read "Test Data"() -> (w343:string[][])
        n151 = for {
          tunnel: w333 -> [_] mode=indexing
          tunnel: ["0"] -> w330 mode=indexing
        }
        n152 = Index Array(array=w343, index (col)=0 ("disabled index (col)")) -> (element=w339:string[])  [unwired: 1 in]
        n153 = local read "Model"() -> (w348:bool)
        n154 = Index Array(array=w339) -> (element #1=w342:string, element #2=w341:string)  [unwired: 2 in]
        n155 = case shown="True" w331 {
          tunnel: "0" -> [w363 w368]
          tunnel: w342 -> [w362 w367]
          tunnel: w341 -> [w361 w366]
          tunnel: [w360 w365] -> w338
          tunnel: w330 -> [w359 w364]
          tunnel: w330 -> [w358 _]
          frame True {
            n156 = Build Array (concatenate)(w362, w361, w363, w363, w359, w363, w363, w358) -> (w360:string[])
          }
          frame False {
            n157 = Build Array (concatenate)(w367, w366, w368, w368, w364) -> (w365:string[])
          }
        }
        n158 = local read "Power OK"() -> (w340:bool)
        n159 = Select(t=w339, s=w340, f=w338) -> (s? t:f=w332:string[])
        n160 = local read "Test Result"() -> (w336:bool)
        n161 = Select(t=w347, s=w348, f=w346) -> (s? t:f=w345:string)
        n162 = call "Data Logger.vi"("PN In"=w345, "Test Result?"=w336, "Error In"=w354, "DB File"=w353, "Model (F-ME74)"=w348, "Test Data In"=w332) -> ("Error Out"=w351:errorcluster, "LBL Data"=w335:T2)  [unwired: 3 in, 1 out]
        "LBL Data" <- w335
        n163 = Not(x=w336) -> (.not. x?=w337:bool)
        n164 = local write "Pass"(w336) -> ()
        n165 = Unbundle By Name(w335) -> ("SN_INT"=w334:i32)
        n166 = local write "Fail"(w337) -> ()
        n167 = control-ref of="Test Data"() -> (w349:refnum<vi>)
        n168 = local write "SN"(w334) -> ()
        n169 = call "Log File.vi"("Error In"=w351, "Model (F-ME74)"=w348, "Test Data table"=w349) -> ("Error Out"=w350:errorcluster)  [unwired: 8 in]
      }
      frame "Print Label" {
        n170 = local read "Test Data"() -> (w381:string[][])
        n171 = local read "LBL Data"() -> (w379:T2)
        n172 = Get Date/Time In Seconds() -> (seconds since 1Jan1904=w393:timestamp)
        n173 = Format Date/Time String(time format string (%c)="%H%M", seconds (now)=w393) -> (date/time string=w391:string)  [unwired: 1 in]
        n174 = call "NGCode.vi"("error in (no error)"=w383, "Test Data"=w381) -> ("error out"=w382:errorcluster, "NG CODE OUT"=w380:string)  [unwired: 8 in]
        n175 = Unbundle(w379) -> ("DT"=w396:string, "SN"=w395:string)  [unwired: 3 out]
        n176 = local read "File Open Reference out"() -> (w394:T1)
        n177 = local read "Test Result"() -> (w386:bool)
        n178 = Bundle(w377, "DT"=w396, "SN"=w395, "date/time string"=w391, "LINECODE"="1", "NG CODE OUT"=w380) -> (w389:T18)  [unwired: 1 in]
        n179 = Bundle By Name(cluster=w379, "PN"=w378, "VPN"=w377) -> (w388:T2)
        n180 = Select(t=TRUE, s=w375, f="ZEBRA PRINT ME74") -> (s? t:f=w370:bool)
        n181 = And(x="Print", y=w370) -> (x .and. y?=w371:bool)
        n182 = case shown="True" w371 {
          tunnel: w382 -> [w404 w413]
          tunnel: [w404 w412] -> w397
          tunnel: w394 -> [_ w411]
          tunnel: w389 -> [_ w410]
          tunnel: w388 -> [_ w409]
          tunnel: w386 -> [_ w408]
          tunnel: w375 -> [_ w407]
          tunnel: [FALSE FALSE] -> w385
          tunnel: [TRUE TRUE] -> w384
          frame False {
          }
          frame True {
            n183 = call "Label PrintOut.vi"("Model (F-ME74)"=w407, "Label Print Pass/Fail (F-Fail)"=w408, "error in (no error)"=w413, "Fail Data"=w410, "Pass Data"=w409, "Labels Reference In"=w411) -> ("error out"=w412:errorcluster)  [unwired: 5 in]
          }
        }
        n184 = Bundle By Name(cluster=w379, "PN"=w378, "VPN"=w377) -> (w376:T2)
        n185 = local write "LBL Data"(w376) -> ()
        n186 = local write "Done"(w384) -> ()
        n187 = local write "Busy"(w385) -> ()
        n188 = Not(x=w386) -> (.not. x?=w387:bool)
        n189 = local write "Pass"(w386) -> ()
        n190 = local write "Fail"(w387) -> ()
      }
      frame "Display Result" {
        n191 = flat-sequence {
          tunnel: w417 -> [w443]
          tunnel: [w443] -> w416
          tunnel: [w438] -> w415
          frame #0 {
            n192 = local read "Test Error"() -> (w440:bool)
            n193 = local read "MCError"() -> (w439:bool)
            n194 = local write "Done"(TRUE) -> ()
            n195 = local write "Busy"(FALSE) -> ()
            n196 = Or(x=w439, y=w440) -> (x .or. y?=w438:bool)
          }
        }
        n197 = Wait (ms)(milliseconds to wait=u32 500) -> ()  [unwired: 1 out]
        n198 = disable-structure shown="Disabled" {
          disable-tunnel: [w425 w437] -> w418
          disable-tunnel: w416 -> [w424 w437]
          disable-tunnel: w415 -> [w423 _]
          frame Disabled {
            n199 = case shown="False" w423 {
              tunnel: [w427 w435] -> w425
              tunnel: w424 -> [w426 w436]
              frame False {
                n200 = local read "Test Result"() -> (w428:bool)
                n201 = case shown="True" w428 {
                  tunnel: w426 -> [w431 w434]
                  tunnel: [w430 w433] -> w427
                  frame False {
                    n202 = local write "Fail"(TRUE ("Pass")) -> ()
                    n203 = call "Fail Result.vi"("error in (no error)"=w431) -> ("error out"=w430:errorcluster)  [unwired: 10 in]
                  }
                  frame True {
                    n204 = local write "Pass"(TRUE ("Pass")) -> ()
                    n205 = call "Pass Result.vi"("error in (no error)"=w434) -> ("error out"=w433:errorcluster)  [unwired: 10 in]
                  }
                }
              }
              frame True {
                n206 = call "Error Result.vi"("error in (no error)"=w436) -> ("error out"=w435:errorcluster)  [unwired: 10 in]
              }
            }
          }
          frame Enabled {
          }
        }
      }
      frame "Quit" {
        n207 = local read "File Open Reference out"() -> (w444:T1)
        n208 = call "Close Labels.vi"("Labels Reference In"=w444) -> ()  [unwired: 10 in, 1 out]
      }
      frame "Calibration" {
        # "Do Speaker Calibration"
        n209 = case shown="True" w464 {
          tunnel: path "D:/Config/ME79ISO40.txt" -> [_ w476]
          tunnel: path "D:/Config/ME74ISO40.txt" -> [w474 _]
          tunnel: [w474 w476] -> w463
          tunnel: w462 -> [_ w475]
          tunnel: w461 -> [w473 _]
          tunnel: [w473 w475] -> w460
          frame False {
            # "ME74"
          }
          frame True {
            # "ME79"
          }
        }
        n210 = flat-sequence {
          tunnel: w457 -> [w471]
          tunnel: [w471] -> w456
          frame #0 {
            n211 = local write "Cal Mic CH"(TRUE ("IAI Cal 2")) -> ()
          }
        }
        n212 = Bundle(w463, w460) -> (w459:cluster{path, path})  [unwired: 1 in]
        n213 = call "Calibration GUI.vi"("error in (no error)"=w456, "Skip Ref Mic"=TRUE, "DB File"=w458, "File"=w459) -> ("error out"=w455:errorcluster)  [unwired: 7 in]
        n214 = flat-sequence {
          tunnel: w455 -> [w469]
          tunnel: [w469] -> w454
          frame #0 {
            n215 = local write "Cal Mic CH"(FALSE ("IAI Cal 2")) -> ()
          }
        }
      }
    }
    n216 = call <vilib>:"Simple Error Handler.vi"("error in (no error)"=w61) -> ("error out"=w70:errorcluster)  [unwired: 4 in, 4 out]
    n217 = Or(x=w65, y="Quit") -> (x .or. y?=w49:bool)
    n218 = call <vilib>:"Clear Errors.vi"("error in (no error)"=w70) -> ("error out"=w69:errorcluster)  [unwired: 5 in, 1 out]
    n219 = Select(t=EnumType."Ready" ("Enum"), s=w61, f=w73) -> (s? t:f=w71:T3)
  }
  n220 = while {
    shift-right: [w480] -> _
    shift-left: u16 0 -> [w482]
    tunnel: w10 -> [_]
    tunnel: "IAI ALARM\nEMERGENCY STOP\nLIGHT CURTAIN ALARM\nCOUNTER FULL\nNO PART SET\nCALIBRATION REQUIRED\nPRESSFIT BUFFER NG" -> [w478]
    stop <- w477 stop-if-true
    # "Alarm Display"
    n221 = Not Equal?(x=w482, y="Alarm") -> (x != y?=w481:bool)
    n222 = Wait Until Next ms Multiple(millisecond multiple=u32 10) -> ()  [unwired: 1 out]
    n223 = case shown="True" w481 {
      tunnel: [w484 w487] -> w480
      tunnel: "Alarm" -> [w484 w487]
      tunnel: w478 -> [_ w486]
      frame False {
      }
      frame True {
        n224 = Number To Boolean Array(number=w487) -> (Boolean array=w489:bool[])
        n225 = for {
          tunnel: w489 -> [w494] mode=indexing
          shift-right: [w491] -> w485
          shift-left: "" -> [w490]
          tunnel: w486 -> [w492]
          i -> [w493]
          n226 = case shown="True" w494 {
            tunnel: w493 -> [_ w501]
            tunnel: w492 -> [_ w500]
            tunnel: w490 -> [w495 w498]
            tunnel: [w495 w499] -> w491
            frame False {
            }
            frame True {
              n227 = Pick Line(multi-line string=w500, line index=w501) -> (output string=w497:string)  [unwired: 1 in]
              n228 = Concatenate Strings(w498, w497, "\r") -> (w499:string)
            }
          }
        }
        "Alarm Display" <- w485
        n229 = global write "Global 1.vi" "Alarm Message"(w485) -> ()
      }
    }
    n230 = global read "Global 1.vi" "QUIT"() -> (w477:bool)
  }
  n231 = while {
    tunnel: w10 -> [_]
    stop <- w502 stop-if-true
    # "PLC Ready Status"
    n232 = global read "Global 1.vi" "QUIT"() -> (w502:bool)
    n233 = call <userlib>:"Periodic Trigger__ogtk.vi"("time (ms)"=u32 1000 ("y")) -> ("Triggered"=w505:bool)  [unwired: 12 in, 2 out]
    n234 = case shown="True" w505 {
      frame False {
      }
      frame True {
        n235 = local read "Ready"() -> (w507:bool)
        n236 = Not(x=w507) -> (.not. x?=→"Ready":bool)
      }
    }
    n237 = Wait (ms)(milliseconds to wait=u32 10) -> ()  [unwired: 1 out]
    n238 = disable-structure shown="Disabled" {
      frame Disabled {
        n239 = call "Date Trigger.vi"("y"=u32 1000) -> ()  [unwired: 11 in]
      }
      frame Enabled {
      }
    }
  }
  n240 = while {
    tunnel: w10 -> [_]
    stop <- w510 stop-if-true
    # "Model Selection"
    n241 = local read "Model"() -> (w509:bool)
    n242 = property on="ME79 MODEL" class="Enum (strict)"("Visible"=w509) -> ()  [unwired: 2 in, 2 out]
    n243 = global read "Global 1.vi" "QUIT"() -> (w510:bool)
    n244 = case shown="True" "Change Model" {
      frame False {
      }
      frame True {
        n245 = call "Model Selection.vi"() -> ()  [unwired: 12 in]
      }
    }
    n246 = Wait (ms)(milliseconds to wait=u32 10) -> ()  [unwired: 1 out]
  }
  n247 = local write "Alarm Display"(w11) -> ()
  n248 = while {
    tunnel: w10 -> [_]
    tunnel: [FALSE ("Open/Close")] -> w25
    tunnel: w11 -> [_]
    stop <- w517 stop-if-true
    # "POP UP"
    n249 = shared-variable "My Computer\\OPC.lvlib\\ErrorDisplay"() -> (w519:bool)  [unwired: 1 in, 1 out]
    n250 = shared-variable "My Computer\\OPC.lvlib\\NGDisplay"() -> (w524:bool)  [unwired: 1 in, 1 out]
    n251 = shared-variable "My Computer\\OPC.lvlib\\OKDisplay"() -> (w531:bool)  [unwired: 1 in, 1 out]
    n252 = shared-variable "My Computer\\OPC.lvlib\\Finished"() -> (w513:bool)  [unwired: 1 in, 1 out]
    n253 = Wait (ms)(milliseconds to wait=u32 10) -> ()  [unwired: 1 out]
    n254 = call <userlib>:"Boolean Trigger__ogtk.vi"("Boolean Input"=w531) -> ("Rising Edge"=w530:bool, "Falling Edge"=w528:bool)  [unwired: 1 in]
    n255 = call <userlib>:"Boolean Trigger__ogtk.vi"("Boolean Input"=w524) -> ("Rising Edge"=w525:bool, "Falling Edge"=w527:bool)  [unwired: 1 in]
    n256 = call <userlib>:"Boolean Trigger__ogtk.vi"("Boolean Input"=w519) -> ("Rising Edge"=w520:bool, "Falling Edge"=w522:bool)  [unwired: 1 in]
    n257 = call <userlib>:"Boolean Trigger__ogtk.vi"("Boolean Input"=w513) -> ("Rising Edge"=w514:bool, "Falling Edge"=w516:bool)  [unwired: 1 in]
    n258 = Or(x=w530, y=w528) -> (x .or. y?=w529:bool)
    n259 = Or(x=w525, y=w527) -> (x .or. y?=w526:bool)
    n260 = Or(x=w520, y=w522) -> (x .or. y?=w521:bool)
    n261 = Or(x=w514, y=w516) -> (x .or. y?=w515:bool)
    n262 = case shown="True" w526 {
      tunnel: w525 -> [_ w537]
      frame False {
      }
      frame True {
        n263 = call "CallPopupDialog.vi"("Open/Close"=w537, "Enum"=enum16{"Finished", "Pass", "Fail", "Error"}."Fail") -> ()  [unwired: 10 in]
      }
    }
    n264 = case shown="True" w529 {
      tunnel: w530 -> [_ w539]
      frame False {
      }
      frame True {
        n265 = call "CallPopupDialog.vi"("Open/Close"=w539, "Enum"=enum16{"Finished", "Pass", "Fail", "Error"}."Pass") -> ()  [unwired: 10 in]
      }
    }
    n266 = case shown="True" w521 {
      tunnel: w520 -> [_ w534]
      frame False {
      }
      frame True {
        n267 = call "CallPopupDialog.vi"("Open/Close"=w534, "Enum"=enum16{"Finished", "Pass", "Fail", "Error"}."Error") -> ()  [unwired: 10 in]
      }
    }
    n268 = case shown="True" w515 {
      tunnel: w514 -> [_ w533]
      frame False {
      }
      frame True {
        n269 = call "CallPopupDialog.vi"("Open/Close"=w533, "Enum"=enum16{"Finished", "Pass", "Fail", "Error"}."Finished") -> ()  [unwired: 10 in]
      }
    }
    n270 = global read "Global 1.vi" "QUIT"() -> (w517:bool)
  }
  n271 = call "CallPopupDialog.vi"("Open/Close"=w25) -> ()  [unwired: 11 in]
  n272 = while {
    tunnel: w10 -> [_]
    stop <- w543 stop-if-true
    # "POPUP BARCODE"
    n273 = local read "LBL Data"() -> (w547:T2)
    n274 = Unbundle(w547) -> ("DT"=w545:string, "SN"=w546:string, "VPN"=w544:string)  [unwired: 2 out]
    n275 = shared-variable "My Computer\\OPC.lvlib\\BarcodeRescan"() -> (w550:bool)  [unwired: 1 in, 1 out]
    n276 = Format Into String(format string="%s %s %s", w546, w545, w544) -> (resulting string=w541:string)  [unwired: 2 in, 1 out]
    n277 = local read "Model"() -> (w540:bool)
    n278 = call <userlib>:"Boolean Trigger__ogtk.vi"("Boolean Input"=w550) -> ("Rising Edge"=w549:bool)  [unwired: 1 in, 1 out]
    n279 = case shown="True" w549 {
      tunnel: w541 -> [_ w554]
      tunnel: w540 -> [_ w551]
      frame False {
      }
      frame True {
        n280 = call "BarcodeScan.vi"("Model ME79? (T-ME79)"=w551, "Barcode In"=w554) -> ("NG"=w552:bool, "OK"=w553:bool)  [unwired: 8 in]
        n281 = shared-variable "My Computer\\OPC.lvlib\\BarcodeOK"(w553) -> ()  [unwired: 1 in, 1 out]
        n282 = shared-variable "My Computer\\OPC.lvlib\\BarcodeNG"(w552) -> ()  [unwired: 1 in, 1 out]
      }
    }
    n283 = global read "Global 1.vi" "QUIT"() -> (w543:bool)
    n284 = Wait (ms)(milliseconds to wait=u32 10) -> ()  [unwired: 1 out]
  }
  n285 = global write "Global 1.vi" "QUIT"(w12) -> ()
